vi "Write Key.vi"(8 "Error In":errorcluster, 10 "Key":string, 11 "Keyable In":refnum<class "Keyable.lvclass">) -> (0 "Error Out":errorcluster, 3 "Keyable Out":refnum<class "Keyable.lvclass">)   [LabVIEW 2018, in "Toolkit.lvlib" / "Tokens.lvlib" / "Keyable.lvclass"]
uses:
  Keyable.lvclass
  Keyable.lvclass/Keyable.ctl
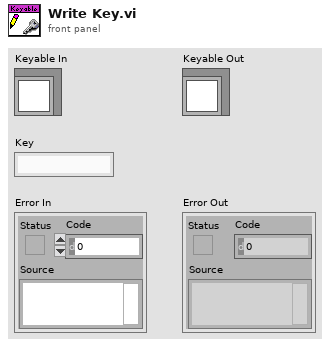
[diagram p1: front panel]
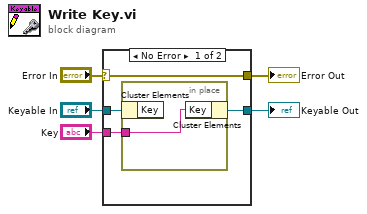
[diagram p0: block diagram]
diagram:
  n1 = case shown="No Error" "Error In" {
    selector: "Error In" -> [w9 w11]
    tunnel: [w9 w11] -> w4
    tunnel: "Keyable In" -> [w8 w12]
    tunnel: "Key" -> [w7 _]
    tunnel: [w6 w12] -> w1
    frame No Error {
      n2 = in-place {
        in-place-border: w7 -> [w10]
        n3 = in-place-cluster #1(w8) -> ()  [unwired: 1 out]
        n4 = in-place-cluster #1("Key"=w10) -> (w6:refnum<class "Keyable.lvclass">)
      }
    }
    frame Error {
    }
  }
  "Error Out" <- w4
  "Keyable Out" <- w1
